vi "ClassPanel.vi"(8 "error in (no error)":errorcluster caption="entrée d'erreur (pas d'erreur)", 11 "KlingerMotor.lvclass":refnum<class "KlingerMotor.lvclass">) -> (0 "error out":errorcluster caption="sortie d'erreur", 3 "KlingerMotor.lvclass Out":refnum<class "KlingerMotor.lvclass">)   [LabVIEW 2019, in "KlingerMotor.lvclass"]
uses:
  KlingerMotor.lvclass
  C:/Programmes Labview/LabScanV1A/DevicesClass/BaseDevice/BaseDevice.lvclass
  <userlib>/KlingerV2/KlingerV2 Params.ctl
  KlingerMotor.lvclass/KlingerMotor.ctl
  BaseDevice/Accessor/GetClassEvent.vi
panel:
  in  "MainProgQ":refnum<queue>
  in  "MainProgQEvent":refnum<user-event>
  out "Nom de l'axe":string
  in  "Enable":bool=TRUE caption="Motor\nEnable"
  in  "Pos_ps":dbl caption="Position (ps)" min=-79999.999 max=79999.999 step=0.001 format="%.3f"
  out "Moving":bool caption="Déplacement\nen cours"
  in  "Axe":u8(ring)=3 items=["W", "X", "Y", "Z"]
  out "NLimit":bool caption="Limite -"
  out "PLimit":bool caption="Limite +"
  in  "Pos_mm":dbl caption="Position (mm)" min=-79999.999 max=79999.999 step=0.001 format="%.4f"
  in  "Stop":bool
  out "Init Program":bool
  # "this MUST labeled with class name"
  # "this MUST be present and labeled \"Stop\""
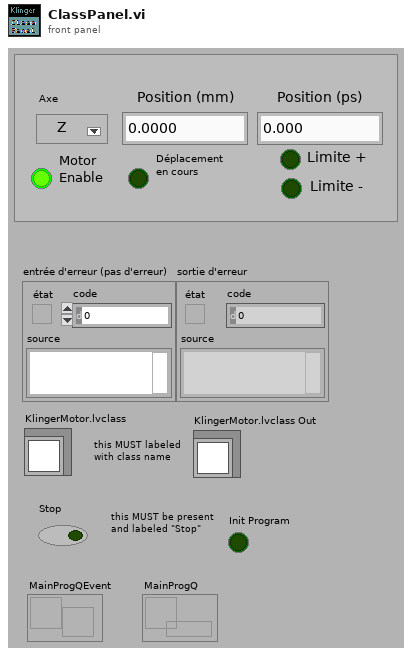
[diagram p1: front panel]
types:
  T1 = typedef "KlingerV2 Params.ctl" = enum16{"Type", "Origine", "Encodeur", "TypeMouv", "FactConv", "Nom", "CorrParams", "KlingCtrlPar", "Speed", "Acc", "Avance", "Tous"}
  T2 = cluster{"Position Ref":refnum<vi>, "Moving Ref":refnum<vi>, "PLimRef":refnum<vi>, "NLimRef":refnum<vi>}
  T3 = cluster{"Minimum":dbl, "Maximum":dbl, "Increment":dbl}
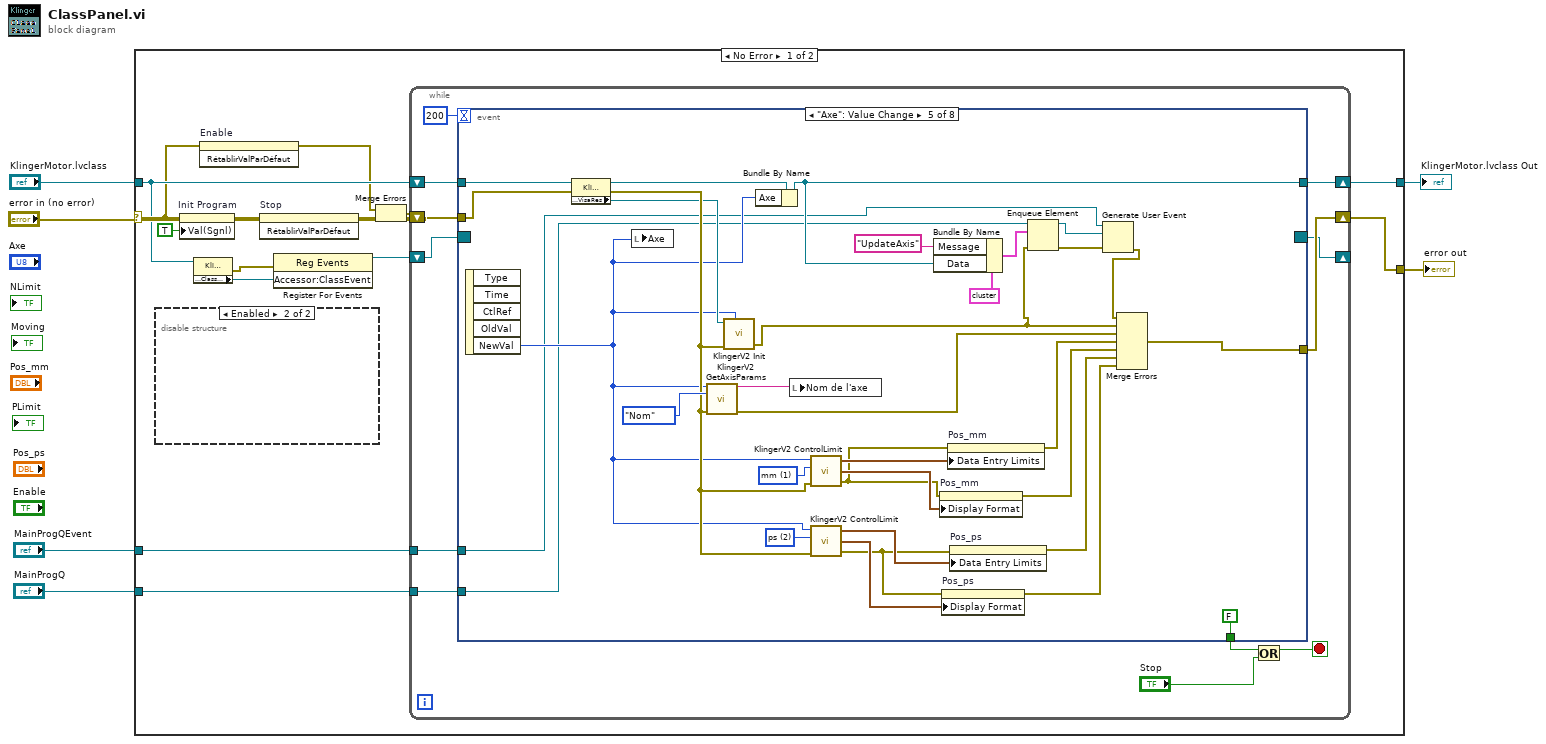
[diagram p0: block diagram]
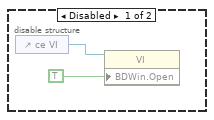
[diagram p2: hidden frame]
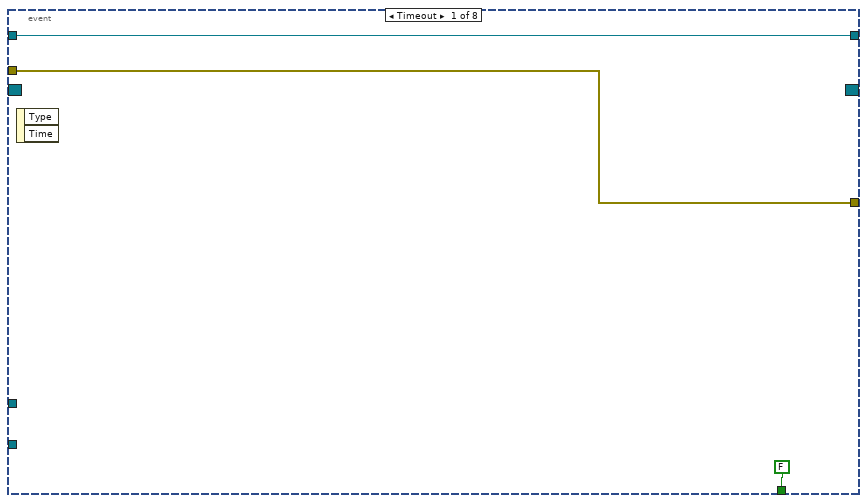
[diagram p3: hidden frame]
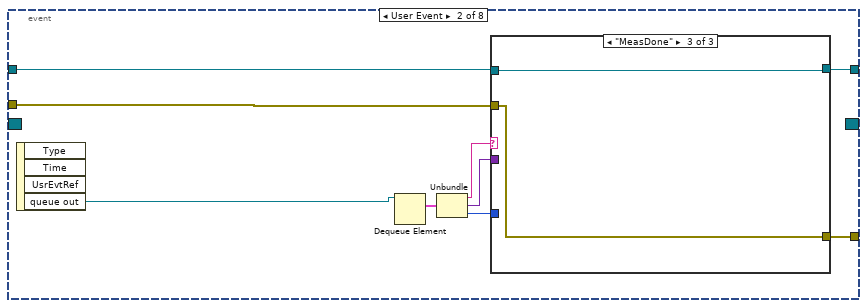
[diagram p4: hidden frame]
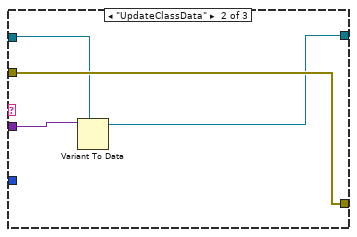
[diagram p6: hidden frame]
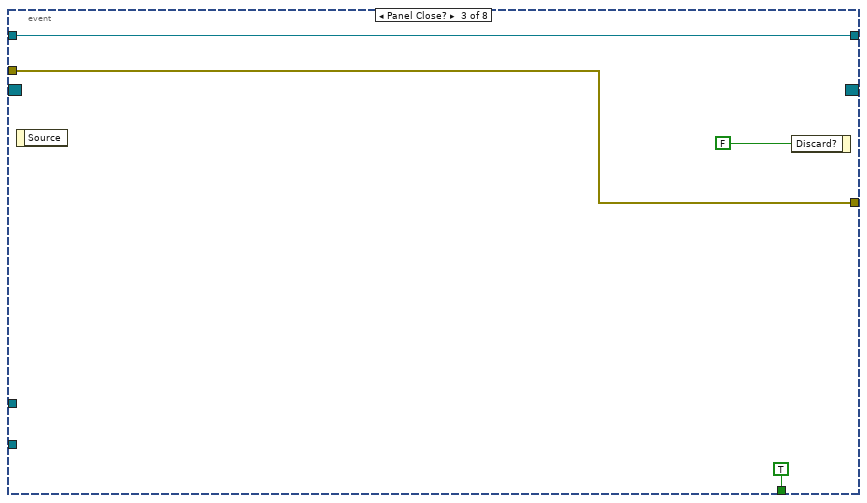
[diagram p7: hidden frame]
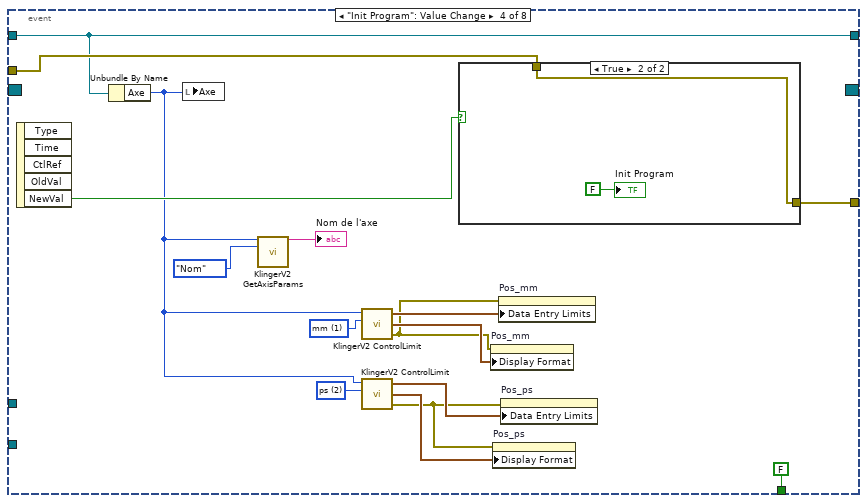
[diagram p8: hidden frame]
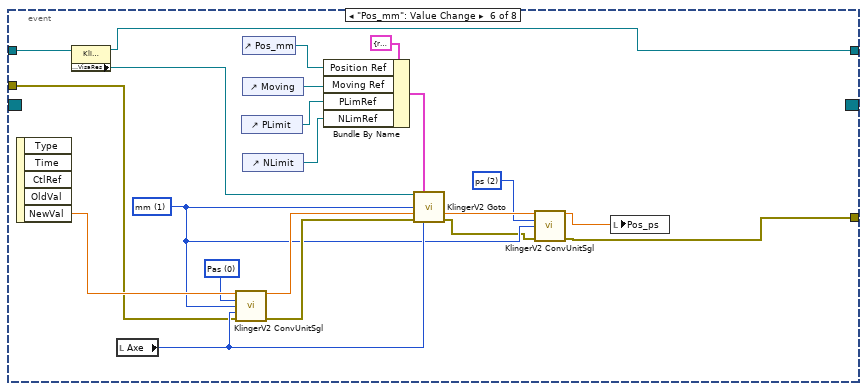
[diagram p10: hidden frame]
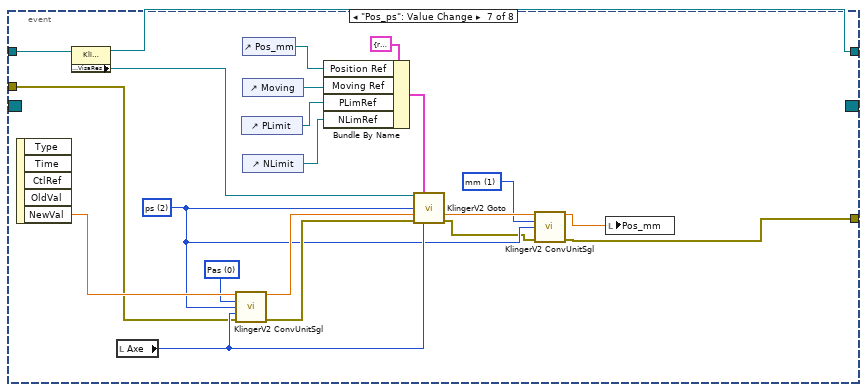
[diagram p11: hidden frame]
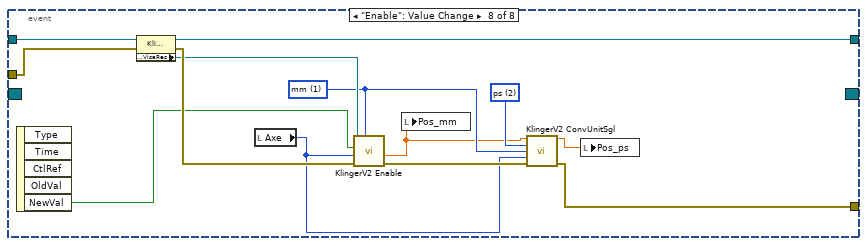
[diagram p12: hidden frame]
diagram:
  n1 = case shown="No Error" "error in (no error)" {
    selector: "error in (no error)" -> [w9 w167]
    tunnel: [w20 w167] -> w5
    tunnel: "KlingerMotor.lvclass" -> [w13 w166]
    tunnel: [w18 w166] -> w3
    tunnel: "MainProgQEvent" -> [w10 _]
    tunnel: "MainProgQ" -> [w11 _]
    frame No Error {
      n2 = disable-structure shown="Enabled" {
        frame Disabled {
          n3 = control-ref of="ce VI"() -> (w22:refnum<vi>)
          n4 = property class="VI"(reference=w22, "BDWin.Open"=TRUE ("Fenêtre du diagramme : ouverte")) -> ()  [unwired: 1 in, 2 out]
        }
        frame Enabled {
        }
      }
      n5 = property on="Init Program" class="Bool (strict)"(error in=w9, "Val(Sgnl)"=TRUE ("Valeur (Signalisation)")) -> (error out=w17:errorcluster)  [unwired: 1 in, 1 out]
      n6 = property class="KlingerMotor.lvclass"(reference=w13) -> (error out=w15:errorcluster, "Accessor:ClassEvent"=w14:refnum<user-event>)  [unwired: 1 in, 1 out]
      n7 = invoke on="Enable" class="Bool (strict)" method="RétablirValParDéfaut"(error in=w9) -> (error out=w7:errorcluster)  [unwired: 2 in, 2 out]
      n8 = invoke on="Stop" class="Bool (strict)" method="RétablirValParDéfaut"(error in=w17) -> (error out=w16:errorcluster)  [unwired: 2 in, 2 out]
      n9 = register-events(error in=w15, w14) -> (reference out=w12:refnum<event-registration>)  [unwired: 1 in, 1 out]
      n10 = Merge Errors(w7, w16) -> (w8:errorcluster)
      n11 = while {
        shift-right: [w32] -> w20
        shift-left: w8 -> [w33]
        shift-right: [w29] -> w18
        shift-left: w13 -> [w31]
        shift-right: [w25] -> _
        shift-left: w12 -> [w26]
        tunnel: w11 -> [w24]
        tunnel: w10 -> [w23]
        stop <- w28 stop-if-true
        n12 = event shown="[4] \"Axe\": Value Change" {
          selector: w26 -> [_ _ _ _ _ _ _ _]
          dyn-events: [_ _ _ _ _ _ _ _] -> w25
          timeout: 200 -> [_ _ _ _ _ _ _ _]
          tunnel: w33 -> [w35 w45 w56 w73 w93 w128 w149 w163]
          tunnel: [w35 w39 w56 w72 w95 w112 w133 w155] -> w32
          tunnel: w31 -> [w36 w46 w55 w70 w91 w125 w146 w165]
          tunnel: [FALSE _ TRUE FALSE FALSE _ _ _] -> w30
          tunnel: [w36 w38 w55 w70 w82 w111 w132 w164] -> w29
          tunnel: w24 -> [_ _ _ _ w81 _ _ _]
          tunnel: w23 -> [_ _ _ _ w80 _ _ _]
          event Timeout {
            n13 = event-data() -> ()  [unwired: 1 in, 2 out]
          }
          event User Event {
            n14 = event-data() -> ("queue out"=w43:refnum<queue>)  [unwired: 1 in, 3 out]
            n15 = Dequeue Element(queue=w43) -> (element=w44:cluster{"Message":string, "Data":variant, i32})  [unwired: 2 in, 3 out]
            n16 = Unbundle(w44) -> ("Message"=w42:string, "Data"=w41:variant, w40:i32)
            n17 = case shown="\"MeasDone\"" w42 {
              tunnel: w45 -> [w48 w52 w53]
              tunnel: w41 -> [_ w51 _]
              tunnel: w46 -> [w47 w50 w54]
              tunnel: [w47 w49 w54] -> w38
              tunnel: [w48 w52 w53] -> w39
              tunnel: w40 -> [_ _ _]
              frame Default {
              }
              frame "UpdateClassData" {
                n18 = Variant To Data(type=w50, Variant=w51) -> (data=w49:refnum<class "KlingerMotor.lvclass">)  [unwired: 1 in, 1 out]
              }
              frame "MeasDone" {
              }
            }
          }
          event Panel Close? {
            n19 = event-data() -> ()  [unwired: 1 in, 1 out]
            n20 = event-data("Discard?"=FALSE ("Rejeter ?")) -> ()  [unwired: 1 in, 1 out]
          }
          event "Init Program": Value Change {
            w64 = u8 1 items=["Pas", "mm", "ps", "Degré (°)"] ("UnitDem")
            w65 = u8 2 items=["Pas", "mm", "ps", "Degré (°)"] ("UnitDem")
            n21 = event-data() -> ("NewVal"=w74:bool)  [unwired: 1 in, 4 out]
            n22 = Unbundle By Name(w70) -> ("Axe"=w61:u8)
            n23 = local write "Axe"(w61) -> ()
            n24 = call <userlib>:"KlingerV2 GetAxisParams.vi"("Axe"=w61, "Param"=KlingerV2_Params."Nom") -> ("Nom de l'axe"=→"Nom de l'axe":string)  [unwired: 4 in, 9 out]
            n25 = call <userlib>:"KlingerV2 ControlLimit.vi"("Axe"=w61, "UnitDem"=w64) -> ("DataRange"=w69:T3, "FormtPrec"=w68:cluster{"Format":u8, "Precision":u8}, "error out"=w62:errorcluster)  [unwired: 3 in]
            n26 = call <userlib>:"KlingerV2 ControlLimit.vi"("Axe"=w61, "UnitDem"=w65) -> ("DataRange"=w67:T3, "FormtPrec"=w66:cluster{"Format":u8, "Precision":u8}, "error out"=w63:errorcluster)  [unwired: 3 in]
            n27 = case shown="True" w74 {
              tunnel: w73 -> [w75 w76]
              tunnel: [w75 w76] -> w72
              frame False {
              }
              frame True {
                "Init Program" <- FALSE
              }
            }
            n28 = property on="Pos_mm" class="NumNb (strict)"(error in=w62, "Display Format"=w68) -> ()  [unwired: 1 in, 2 out]
            n29 = property on="Pos_ps" class="NumNb (strict)"(error in=w63, "Display Format"=w66) -> ()  [unwired: 1 in, 2 out]
            n30 = property on="Pos_mm" class="NumNb (strict)"(error in=w62, "Data Entry Limits"=w69) -> ()  [unwired: 1 in, 2 out]
            n31 = property on="Pos_ps" class="NumNb (strict)"(error in=w63, "Data Entry Limits"=w67) -> ()  [unwired: 1 in, 2 out]
          }
          event "Axe": Value Change {
            w104 = u8 1 items=["Pas", "mm", "ps", "Degré (°)"] ("UnitDem")
            w105 = u8 2 items=["Pas", "mm", "ps", "Degré (°)"] ("UnitDem")
            n32 = event-data() -> ("NewVal"=w86:u8)  [unwired: 1 in, 4 out]
            n33 = property class="KlingerMotor.lvclass"(reference=w91, error in=w93) -> (reference out=w87:refnum<class "KlingerMotor.lvclass">, error out=w92:errorcluster, "Accessor:VisaRes"=w90:refnum<visa-resource-name>)
            n34 = local write "Axe"(w86) -> ()
            n35 = call <userlib>:"KlingerV2 GetAxisParams.vi"("Axe"=w86, "Param"=KlingerV2_Params."Nom", "error in"=w92) -> ("Nom de l'axe"=w94:string, "error out"=w100:errorcluster)  [unwired: 3 in, 8 out]
            n36 = call <userlib>:"KlingerV2 Init.vi"("VISA_Res"=w90, "error in"=w92, "Axe"=w86) -> ("error out"=w79:errorcluster)  [unwired: 2 in, 2 out]
            n37 = Bundle By Name(cluster=w87, "Axe"=w86) -> (w82:refnum<class "KlingerMotor.lvclass">)
            n38 = local write "Nom de l'axe"(w94) -> ()
            n39 = call <userlib>:"KlingerV2 ControlLimit.vi"("Axe"=w86, "UnitDem"=w104, "error in"=w92) -> ("DataRange"=w109:T3, "FormtPrec"=w108:cluster{"Format":u8, "Precision":u8}, "error out"=w102:errorcluster)  [unwired: 2 in]
            n40 = call <userlib>:"KlingerV2 ControlLimit.vi"("Axe"=w86, "UnitDem"=w105, "error in"=w92) -> ("DataRange"=w107:T3, "FormtPrec"=w106:cluster{"Format":u8, "Precision":u8}, "error out"=w103:errorcluster)  [unwired: 2 in]
            n41 = Bundle By Name(cluster=cluster{"Message":string, "Data":variant, i32} {"Message"="", "Data"=variant, 0} ("élément"), "Message"="UpdateAxis", "Data"=w82) -> (w84:cluster{"Message":string, "Data":variant, i32})
            n42 = property on="Pos_mm" class="NumNb (strict)"(error in=w102, "Display Format"=w108) -> (error out=w98:errorcluster)  [unwired: 1 in, 1 out]
            n43 = property on="Pos_ps" class="NumNb (strict)"(error in=w103, "Display Format"=w106) -> (error out=w96:errorcluster)  [unwired: 1 in, 1 out]
            n44 = property on="Pos_mm" class="NumNb (strict)"(error in=w102, "Data Entry Limits"=w109) -> (error out=w99:errorcluster)  [unwired: 1 in, 1 out]
            n45 = property on="Pos_ps" class="NumNb (strict)"(error in=w103, "Data Entry Limits"=w107) -> (error out=w97:errorcluster)  [unwired: 1 in, 1 out]
            n46 = Enqueue Element(queue=w81, element=w84, error in (no error)=w79) -> (queue out=w88:refnum<queue>, error out=w89:errorcluster)  [unwired: 1 in, 1 out]
            n47 = Generate User Event(user event=w80, event data cluster=w88, error in=w89) -> (error out=w78:errorcluster)  [unwired: 1 in, 1 out]
            n48 = Merge Errors(w78, w79, w100, w99, w98, w97, w96) -> (w95:errorcluster)
          }
          event "Pos_mm": Value Change {
            w115 = u8 2 items=["Pas", "mm", "ps", "Degré (°)"] ("UnitDem")
            w116 = u8 1 items=["Pas", "mm", "ps", "Degré (°)"] ("UnitAct")
            w130 = u8 0 items=["Pas", "mm", "ps", "Degré (°)"] ("UnitDem")
            n49 = event-data() -> ("NewVal"=w131:dbl)  [unwired: 1 in, 4 out]
            n50 = property class="KlingerMotor.lvclass"(reference=w125) -> (reference out=w111:refnum<class "KlingerMotor.lvclass">, "Accessor:VisaRes"=w124:refnum<visa-resource-name>)  [unwired: 1 in, 1 out]
            n51 = local read "Axe"() -> (w129:u8)
            n52 = call <userlib>:"KlingerV2 ConvUnitSgl.vi"("ParamAct"=w131, "UnitDem"=w130, "UnitAct"=w116, "Axe"=w129, "error in"=w128) -> ("ParamDem"=w127:dbl, "error out"=w126:errorcluster)  [unwired: 9 in]
            n53 = control-ref of="PLimit"() -> (w119:refnum<vi>)
            n54 = control-ref of="Pos_mm"() -> (w120:refnum<vi>)
            n55 = control-ref of="Moving"() -> (w121:refnum<vi>)
            n56 = control-ref of="NLimit"() -> (w118:refnum<vi>)
            n57 = Bundle By Name(cluster=T2 {"Position Ref"=refnum, "Moving Ref"=refnum, "PLimRef"=refnum, "NLimRef"=refnum} ("Ctrl Refs"), "Position Ref"=w120, "Moving Ref"=w121, "PLimRef"=w119, "NLimRef"=w118) -> (w122:T2)
            n58 = call <userlib>:"KlingerV2 Goto.vi"("VISA Rsrc"=w124, "Ctrl Refs"=w122, "UnitDem"=w116, "PosDem"=w127, "error in"=w126, "Axe"=w129) -> ("Position Out"=w117:dbl, "error out"=w113:errorcluster)  [unwired: 3 in, 5 out]
            n59 = call <userlib>:"KlingerV2 ConvUnitSgl.vi"("ParamAct"=w117, "UnitDem"=w115, "UnitAct"=w116, "error in"=w113) -> ("ParamDem"=w114:dbl, "error out"=w112:errorcluster)  [unwired: 10 in]
            n60 = local write "Pos_ps"(w114) -> ()
          }
          event "Pos_ps": Value Change {
            w136 = u8 1 items=["Pas", "mm", "ps", "Degré (°)"] ("UnitDem")
            w137 = u8 2 items=["Pas", "mm", "ps", "Degré (°)"] ("UnitAct")
            w151 = u8 0 items=["Pas", "mm", "ps", "Degré (°)"] ("UnitDem")
            n61 = event-data() -> ("NewVal"=w152:dbl)  [unwired: 1 in, 4 out]
            n62 = property class="KlingerMotor.lvclass"(reference=w146) -> (reference out=w132:refnum<class "KlingerMotor.lvclass">, "Accessor:VisaRes"=w145:refnum<visa-resource-name>)  [unwired: 1 in, 1 out]
            n63 = local read "Axe"() -> (w150:u8)
            n64 = call <userlib>:"KlingerV2 ConvUnitSgl.vi"("ParamAct"=w152, "UnitDem"=w151, "UnitAct"=w137, "Axe"=w150, "error in"=w149) -> ("ParamDem"=w148:dbl, "error out"=w147:errorcluster)  [unwired: 9 in]
            n65 = control-ref of="PLimit"() -> (w140:refnum<vi>)
            n66 = control-ref of="Pos_mm"() -> (w141:refnum<vi>)
            n67 = control-ref of="Moving"() -> (w142:refnum<vi>)
            n68 = control-ref of="NLimit"() -> (w139:refnum<vi>)
            n69 = Bundle By Name(cluster=T2 {"Position Ref"=refnum, "Moving Ref"=refnum, "PLimRef"=refnum, "NLimRef"=refnum} ("Ctrl Refs"), "Position Ref"=w141, "Moving Ref"=w142, "PLimRef"=w140, "NLimRef"=w139) -> (w143:T2)
            n70 = call <userlib>:"KlingerV2 Goto.vi"("VISA Rsrc"=w145, "Ctrl Refs"=w143, "UnitDem"=w137, "PosDem"=w148, "error in"=w147, "Axe"=w150) -> ("Position Out"=w138:dbl, "error out"=w134:errorcluster)  [unwired: 3 in, 5 out]
            n71 = call <userlib>:"KlingerV2 ConvUnitSgl.vi"("ParamAct"=w138, "UnitDem"=w136, "UnitAct"=w137, "error in"=w134) -> ("ParamDem"=w135:dbl, "error out"=w133:errorcluster)  [unwired: 10 in]
            n72 = local write "Pos_mm"(w135) -> ()
          }
          event "Enable": Value Change {
            w159 = u8 2 items=["Pas", "mm", "ps", "Degré (°)"] ("UnitDem")
            w157 = u8 1 items=["Pas", "mm", "ps", "Degré (°)"] ("UnitDem")
            n73 = event-data() -> ("NewVal"=w161:bool)  [unwired: 1 in, 4 out]
            n74 = property class="KlingerMotor.lvclass"(reference=w165, error in=w163) -> (reference out=w164:refnum<class "KlingerMotor.lvclass">, error out=w162:errorcluster, "Accessor:VisaRes"=w160:refnum<visa-resource-name>)
            n75 = local read "Axe"() -> (w153:u8)
            n76 = call <userlib>:"KlingerV2 Enable.vi"("UnitDem"=w157, "error in"=w162, "Axe"=w153, "Enable"=w161, "VISA Rsrc"=w160) -> ("error out"=w158:errorcluster, "Position"=w154:dbl)  [unwired: 2 out]
            n77 = local write "Pos_mm"(w154) -> ()
            n78 = call <userlib>:"KlingerV2 ConvUnitSgl.vi"("ParamAct"=w154, "UnitDem"=w159, "UnitAct"=w157, "Axe"=w153, "error in"=w158) -> ("ParamDem"=w156:dbl, "error out"=w155:errorcluster)  [unwired: 9 in]
            n79 = local write "Pos_ps"(w156) -> ()
          }
        }
        n80 = Or(x=w30, y="Stop") -> (x .or. y?=w28:bool)
      }
    }
    frame Error {
    }
  }
  "error out" <- w5
  "KlingerMotor.lvclass Out" <- w3
